vi "Latch.vi"(11 "Input":bool) -> (3 "Output":bool)   [LabVIEW 2016]
doc: "When input becomes true output stays true even if input goes false again"
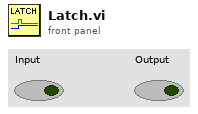
[diagram p1: front panel]
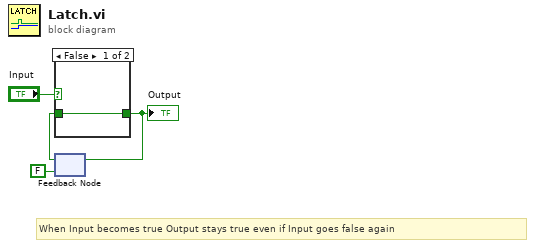
[diagram p0: block diagram]
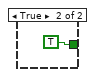
[diagram p2: hidden frame]
diagram:
  # "When Input becomes true Output stays true even if Input goes false again"
  n1 = feedback #1(FALSE ("Output")) -> (w3:bool)
  n2 = case shown="False" "Input" {
    tunnel: [w5 TRUE ("Output")] -> w2
    tunnel: w3 -> [w5 _]
    frame False {
    }
    frame True {
    }
  }
  "Output" <- w2
  n3 = feedback-in #1(w2) -> ()
